vi "classes.vi"(0 "HB_Factory":refnum<class "HB_DeviceFactory.lvclass">, 1 "className":string, 5 "error in (no error)":errorcluster) -> (14 "dup HB_Factory":refnum<class "HB_DeviceFactory.lvclass">, 16 "Object":refnum<class>, 19 "error out":errorcluster)   [LabVIEW 2009, in "HB_Device_Examples.lvlib" / "HB_DeviceFactory.lvclass"]
doc: "This dynamaic dispatch VI contains constant objects of all classes that can be produced by HB_Factory.\n\nChild classes can override it to define additional classes."
uses:
  HB_DeviceFactory.lvclass
  NInstrSim.lvclass
  Visitors/NInstrSim_ConfigureVDCRange/NInstrSim_ConfigureVDCRange.lvclass
  Visitors/NInstrSim_ConfigureWaveformFormat/NInstrSim_ConfigureWaveformFormat.lvclass
  Visitors/NInstrSim_ConfigureWaveformType/NInstrSim_ConfigureWaveformType.lvclass
  Visitors/NInstrSim_ReadDCMeasurement/NInstrSim_ReadDCMeasurement.lvclass
  Visitors/NInstrSim_ReadWaveform/NInstrSim_ReadWaveform.lvclass
  Visitors/NInstrSim_ReadStatus/NInstrSim_ReadStatus.lvclass
  HB_Factory/HB_Factory.lvclass
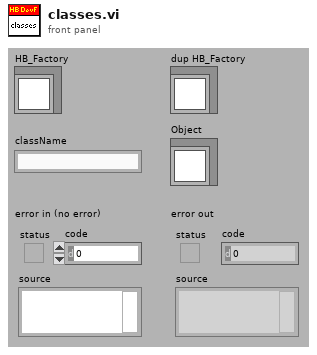
[diagram p1: front panel]
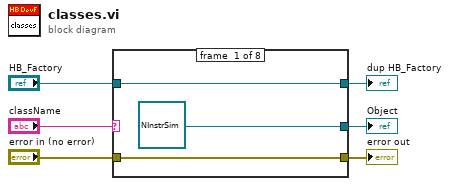
[diagram p0: block diagram]
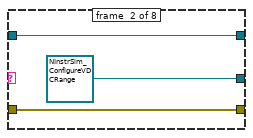
[diagram p2: hidden frame]
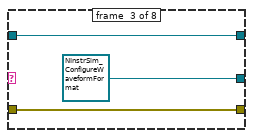
[diagram p3: hidden frame]
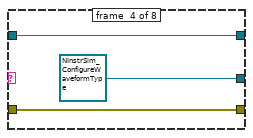
[diagram p4: hidden frame]
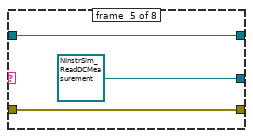
[diagram p5: hidden frame]
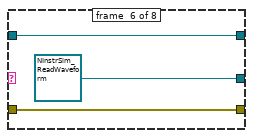
[diagram p6: hidden frame]
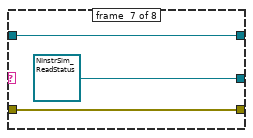
[diagram p7: hidden frame]
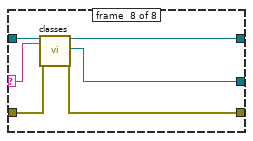
[diagram p8: hidden frame]
diagram:
  n1 = case shown="\"NInstrSim\"" "className" {
    selector: "className" -> [_ _ _ _ _ _ _ w28]
    tunnel: "HB_Factory" -> [w9 w11 w14 w18 w21 w24 w27 w33]
    tunnel: "error in (no error)" -> [w8 w10 w13 w17 w20 w23 w26 w32]
    tunnel: [w9 w11 w14 w18 w21 w24 w27 w31] -> w4
    tunnel: [refnum<class "NInstrSim.lvclass"> refnum ("HB_HGF_Test.lvlib:NInstrSim.lvclass") refnum<class "NInstrSim_ConfigureVDCRange.lvclass"> refnum ("HB_HGF_Test.lvlib:NInstrSim_ConfigureVDCRange.lvclass") refnum<class "NInstrSim_ConfigureWaveformFormat.lvclass"> refnum ("HB_HGF_Test.lvlib:NInstrSim_ConfigureWaveformFormat.lvclass") refnum<class "NInstrSim_ConfigureWaveformType.lvclass"> refnum ("HB_HGF_Test.lvlib:NInstrSim_ConfigureWaveformType.lvclass") refnum<class "NInstrSim_ReadDCMeasurement.lvclass"> refnum ("HB_HGF_Test.lvlib:NInstrSim_ReadDCMeasurement.lvclass") refnum<class "NInstrSim_ReadWaveform.lvclass"> refnum ("HB_HGF_Test.lvlib:NInstrSim_ReadWaveform.lvclass") refnum<class "NInstrSim_ReadStatus.lvclass"> refnum ("HB_HGF_Test.lvlib:NInstrSim_ReadStatus.lvclass") w30] -> w3
    tunnel: [w8 w10 w13 w17 w20 w23 w26 w29] -> w2
    frame #0 {
    }
    frame #1 {
    }
    frame #2 {
    }
    frame #3 {
    }
    frame #4 {
    }
    frame #5 {
    }
    frame #6 {
    }
    frame #7 {
      n2 = call-parent "classes.vi"("HB_Factory"=w33, "className"=w28, "error in (no error)"=w32) -> ("dup HB_Factory"=w31:refnum<class "HB_DeviceFactory.lvclass">, "Object"=w30:refnum<class>, "error out"=w29:errorcluster)  [unwired: 14 out]
    }
  }
  "error out" <- w2
  "dup HB_Factory" <- w4
  "Object" <- w3
